vi "How to change Port.vi"   [LabVIEW 2018]
uses:
  Spels.AutomationTools.RemoteFunctionalControlService.dll
  Spels.AutomationTools.Utility.Wcf.dll
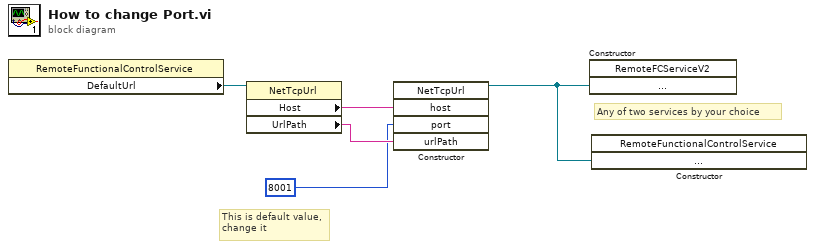
[diagram p0: block diagram]
diagram:
  # "This is default value,\nchange it"
  # "Any of two services by your choice"
  n1 = property class="RemoteFunctionalControlService"() -> ("DefaultUrl"=w5:refnum<k24>)  [unwired: 2 in, 2 out]
  n2 = property class="NetTcpUrl"(reference=w5) -> ("Host"=w4:string, "UrlPath"=w3:string)  [unwired: 1 in, 2 out]
  n3 = constructor class="NetTcpUrl"("host"=w4, "port"=u32 8001, "urlPath"=w3) -> (reference out=w1:refnum<k24>)  [unwired: 3 in, 5 out]
  n4 = constructor class="RemoteFCServiceV2"("serviceUrl"=w1) -> ()  [unwired: 3 in, 4 out]
  n5 = constructor class="RemoteFunctionalControlService"("serviceUrl"=w1) -> ()  [unwired: 3 in, 4 out]
